vi "patientsbtnController.vi"(7 "state":enum16{"Init", "disable", "enable"}(ring), 8 "error in (no error)":errorcluster caption="에러 입력(에러 없음)", 9 "버튼개수":i32=3, 10 "2dArray":string[][](table), 11 "Controls[]":refnum<vi>[](array[refnum])) -> (0 "error out":errorcluster caption="에러 출력")   [LabVIEW 2019]
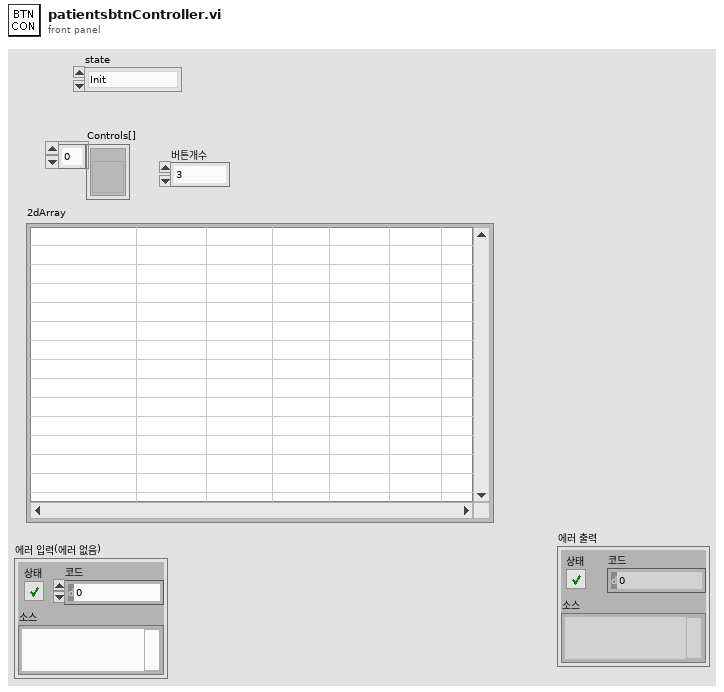
[diagram p1: front panel]
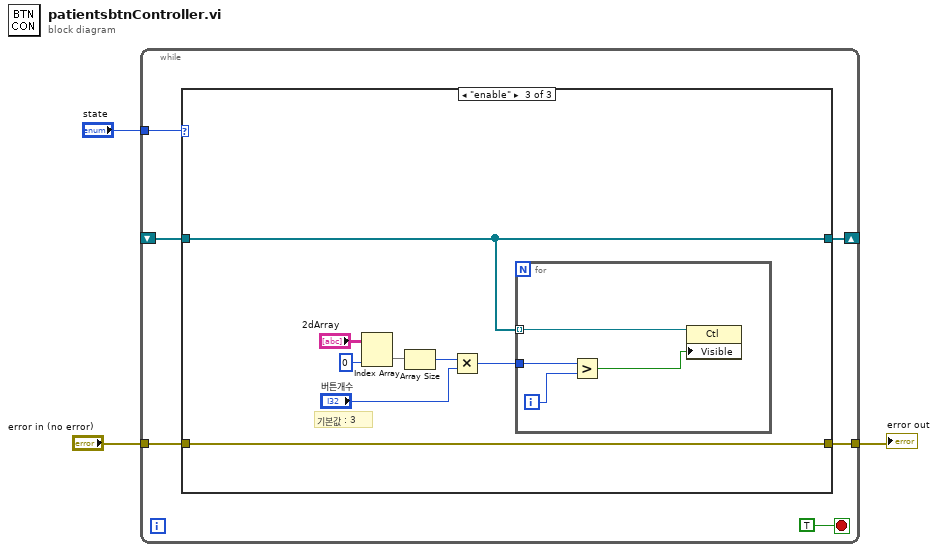
[diagram p0: block diagram]
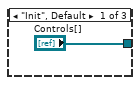
[diagram p2: hidden frame]
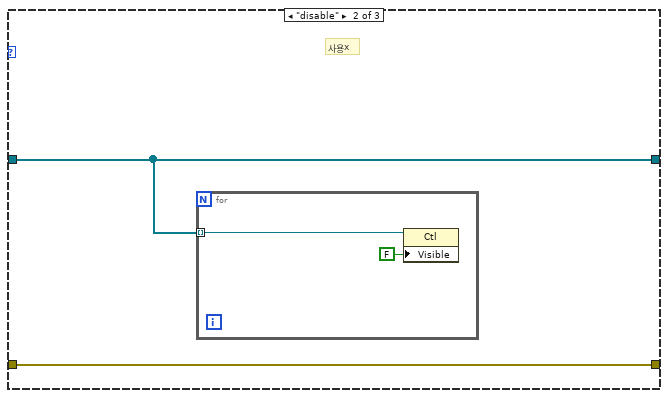
[diagram p3: hidden frame]
diagram:
  n1 = while {
    tunnel: "state" -> [w9]
    shift-right: [w8] -> _
    shift-left: _ -> [w7]
    tunnel: "error in (no error)" -> [w5]
    tunnel: [w4] -> w1
    stop <- TRUE stop-if-true
    n2 = case shown="\"enable\"" w9 {
      tunnel: ["Controls[]" w12 w21] -> w8
      tunnel: w7 -> [_ w12 w21]
      tunnel: w5 -> [_ w11 w22]
      tunnel: [_ w11 w22] -> w4
      frame "Init", Default {
      }
      frame "disable" {
        # "사용x"
        n3 = for {
          tunnel: w12 -> [w14] mode=indexing
          n4 = property class="Ctl"(reference=w14, "Visible"=FALSE ("보이기")) -> ()  [unwired: 1 in, 2 out]
        }
      }
      frame "enable" {
        # "기본값 : 3"
        n5 = Index Array(array="2dArray", index (col)=0 ("비활성화된 인덱스 (열)")) -> (element=w18:string[])  [unwired: 1 in]
        n6 = Array Size(array=w18) -> (size(s)=w17:i32)
        n7 = Multiply(x=w17, y="버튼개수") -> (x*y=w16:i32)
        n8 = for {
          tunnel: w21 -> [w26] mode=indexing
          tunnel: w16 -> [w25]
          i -> [w24]
          n9 = Greater?(x=w25, y=w24) -> (0:w23:bool)
          n10 = property class="Ctl"(reference=w26, "Visible"=w23) -> ()  [unwired: 1 in, 2 out]
        }
      }
    }
  }
  "error out" <- w1
